vi "generador.vi"() -> ()   [LabVIEW 2017]
uses:
  <vilib>/measure/NI_MABase.lvlib
panel:
  in  "stop":bool
  in  "device name":tag="myDAQ1"
  in  "input cluster":T1={"amplitude"=2.0, "frequency"=10.0, "square wave duty cycle (%)"=50.0, "reset signal"=FALSE, "signal type"=enum."Sine Wave", "phase"=0.0} {"phase" format="%.2p"; "square wave duty cycle (%)" format="%0.2f"; "frequency" format="%0.2p"; "amplitude" min=0.0 max=5.0 scale=0.0..5.0}
  in  "Desviación\nEstandar":dbl=1.0 format="%.2p"
  out "data 2":waveform(dbl)(graph) caption="data"
  in  "sampling info":cluster{"Fs":dbl, "#s":dbl}={"Fs"=1000.0, "#s"=1000.0} {"Fs" format="%.2p"}
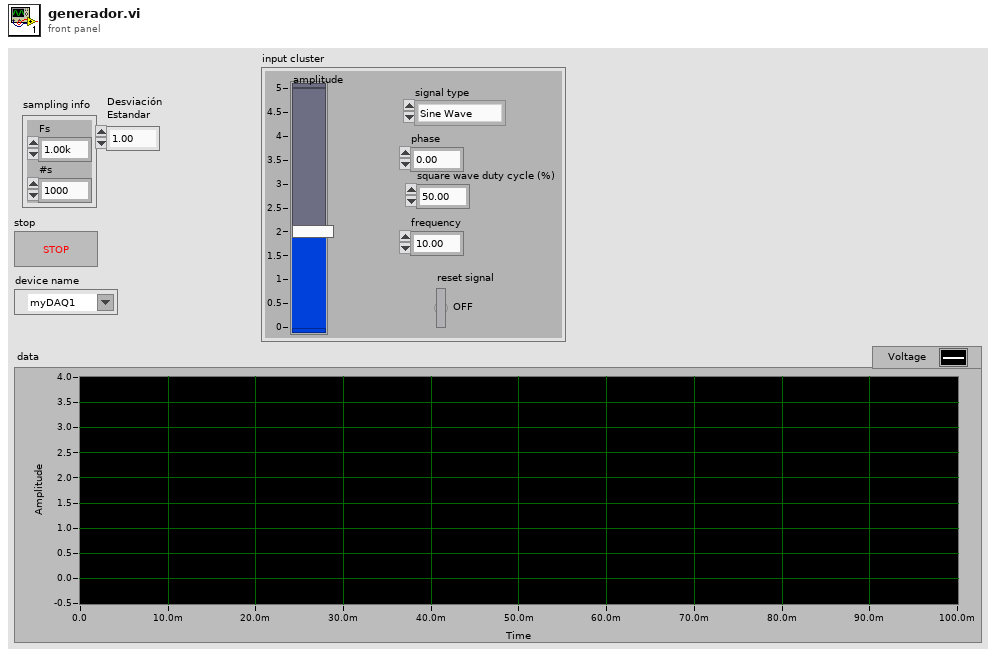
[diagram p1: front panel]
types:
  T1 = cluster{"amplitude":dbl, "frequency":dbl, "square wave duty cycle (%)":dbl, "reset signal":bool, "signal type":enum16{"Sine Wave", "Triangle Wave", "Square Wave", "Sawtooth Wave"}, "phase":dbl}
  T2 = enum16{"Sine Wave", "Triangle Wave", "Square Wave", "Sawtooth Wave"}
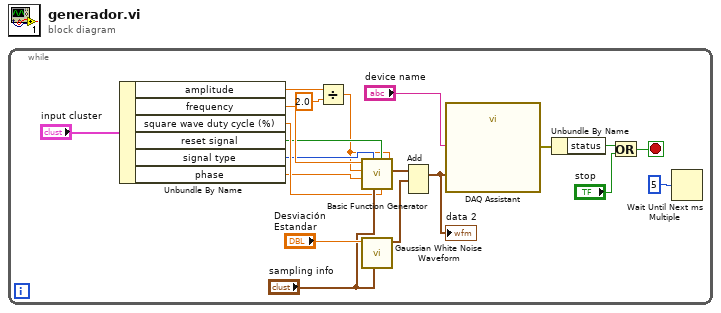
[diagram p0: block diagram]
diagram:
  n1 = while {
    stop <- w12 stop-if-true
    n2 = Unbundle By Name("input cluster") -> ("amplitude"=w3:dbl, "frequency"=w8:dbl, "square wave duty cycle (%)"=w7:dbl, "reset signal"=w6:bool, "signal type"=w5:T2, "phase"=w4:dbl)
    n3 = Divide(x=w3, y=2.0) -> (x/y=w2:dbl)
    n4 = call <vilib>:"Basic Function Generator.vi"("offset"=w2, "square wave duty cycle (%)"=w7, "reset signal"=w6, "sampling info"="sampling info", "signal type"=w5, "phase"=w4, "amplitude"=w2, "frequency"=w8) -> ("signal out"=w17:waveform(dbl))  [unwired: 1 in, 2 out]
    n5 = call <vilib>:"Gaussian White Noise Waveform.vi"("sampling info"="sampling info", "standard deviation"="Desviación\nEstandar") -> ("signal out"=w16:waveform(dbl))  [unwired: 8 in, 1 out]
    n6 = Add(1:w16, 2:w17) -> (0:w14:waveform(dbl))  [unwired: 1 in, 1 out]
    "data 2" <- w14
    n7 = call "DAQ Assistant"("data"=w14, "device name"="device name") -> ("error out"=w13:errorcluster)  [unwired: 16 in, 1 out]
    n8 = Unbundle By Name(w13) -> ("status"=w9:bool)
    n9 = Or(x=w9, y="stop") -> (x .or. y?=w12:bool)
    n10 = Wait Until Next ms Multiple(millisecond multiple=u32 5) -> ()  [unwired: 1 out]
  }
